vi "Acquire Image.vi"(8 "Error In":errorcluster, 10 "File Path":path, 11 "Acquisition Memory":T1[](array[typedef])) -> (0 "Error Out":errorcluster, 1 "Source Image":T1, 2 "HSL Image":T1, 3 "Pre-processed Image":T1, 5 "histogram":u32[](array[numeric]))   [LabVIEW 2018]
uses:
  <vilib>/vision/Image Controls.llb/IMAQ Image.ctl
  <vilib>/vision/NI_Vision_Development_Module.lvlib
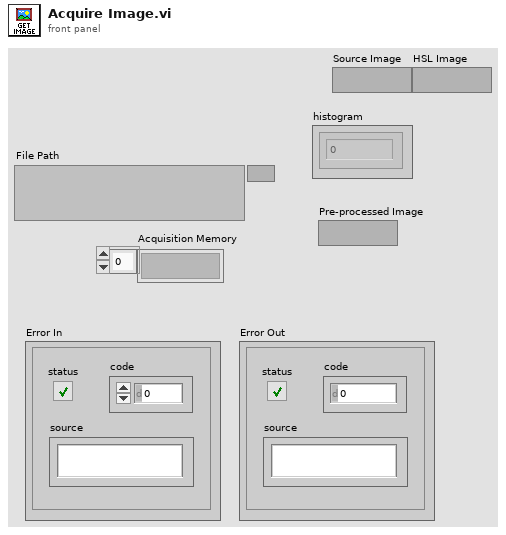
[diagram p1: front panel]
types:
  T1 = typedef "IMAQ Image.ctl" = refnum<image>
  T2 = typedef "Image Type" = u32
  T3 = cluster{"histogram":u32[], "Minimal Value":sgl, "Maximal Value":sgl, "Starting Value":sgl, "Interval Width":sgl, "Mean Value":sgl, "Standard  Variation":sgl, "Area (pixels)":i32}
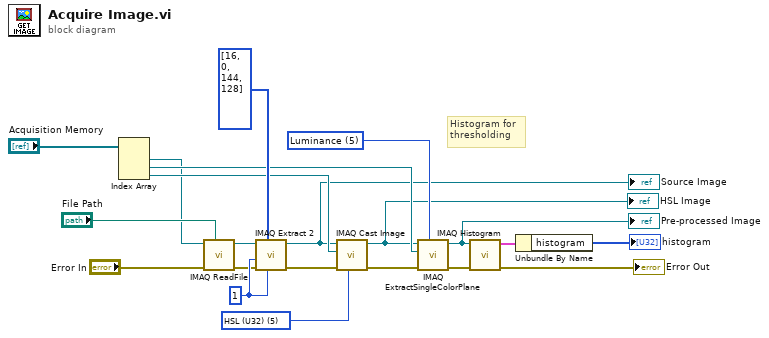
[diagram p0: block diagram]
diagram:
  w11 = 5 items=["Red", "Green", "Blue", "Hue", "Saturation", "Luminance", "Value", "Intensity"] ("Color Plane")
  w15 = T2 5 items=["Grayscale (U8)", "Grayscale (I16)", "Grayscale (SGL)", "Complex (CSG)", "RGB (U32)", "HSL (U32)", "RGB (U64)", "Grayscale (U16)"] ("Image Type")
  w20 = 1 ("Y Step Size")
  # "Histogram for\nthresholding"
  n1 = Index Array(array="Acquisition Memory") -> (element #1=w6:T1, element #2=w10:T1, element #3=w7:T1)  [unwired: 3 in]
  n2 = call "IMAQ ReadFile"("File Path"="File Path", "error in (no error)"="Error In", "Image"=w6) -> ("error out"=w14:errorcluster, "Image Out"=w13:T1)  [unwired: 4 in, 3 out]
  n3 = call "IMAQ Extract 2"("Y Step Size"=w20, "Optional Rectangle"=i32[] [16, 0, 144, 128], "error in (no error)"=w14, "X Step Size"=w20, "Image Src"=w13) -> ("error out"=w4:errorcluster, "Image Dst Out"=w5:T1)  [unwired: 5 in]
  "Source Image" <- w5
  n4 = call "IMAQ Cast Image"("Image Type"=w15, "error in (no error)"=w4, "Image Dst"=w7, "Image Src"=w5) -> ("error out"=w12:errorcluster, "Image Dst Out"=w3:T1)  [unwired: 6 in]
  "HSL Image" <- w3
  n5 = call "IMAQ ExtractSingleColorPlane"("Color Plane"=w11, "error in (no error)"=w12, "Image Dst"=w10, "Image Src"=w3) -> ("error out"=w8:errorcluster, "Image Dst Out"=w9:T1)  [unwired: 6 in]
  "Pre-processed Image" <- w9
  n6 = call "IMAQ Histogram"("error in (no error)"=w8, "Image"=w9) -> ("error out"=→"Error Out":errorcluster, "Histogram Report"=w18:T3)  [unwired: 8 in]
  n7 = Unbundle By Name(w18) -> ("histogram"=→"histogram":u32[])
